vi "Close VISA Resource.vi"(8 "error in (no error)":errorcluster, 11 "Connection Info in":T1) -> (0 "error out":errorcluster)   [LabVIEW 2020, in "plugin_flodx_ph_probe.lvlib" / "plugin.lvlib" / "Instrument Manager.lvlib"]
doc: "Close the VISA resource connection. Calls mock drivers if symbol NO_DRIVER == 1."
uses:
  Instrument Manager.lvlib
  connection_info/Connection Info.ctl
  mock_driver/mock_driver.lvlib
  <instrlib>/RxnRover/FloDx Ph Probe Driver/driver_flodx_ph_probe.lvlib
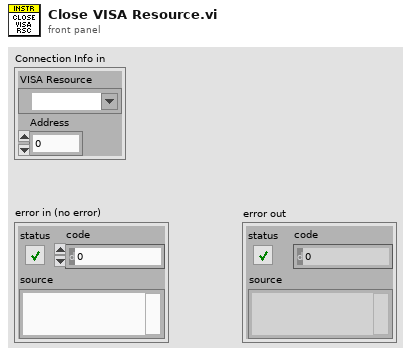
[diagram p1: front panel]
types:
  T1 = typedef "plugin_flodx_ph_probe.lvlib/plugin.lvlib/Instrument Manager.lvlib/Connection Info.ctl" = cluster{"VISA Resource":refnum<visa-resource-name>, "Address":u8}
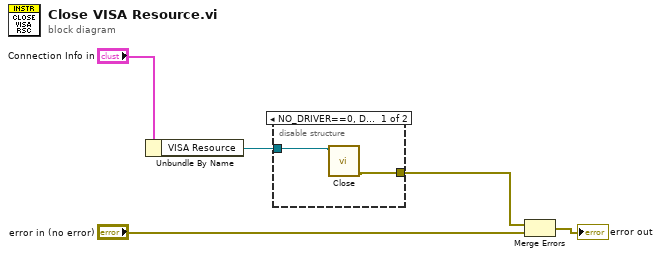
[diagram p0: block diagram]
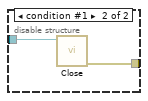
[diagram p2: hidden frame]
diagram:
  n1 = Unbundle By Name("Connection Info in") -> ("VISA Resource"=w1:refnum<visa-resource-name>)
  n2 = disable-structure shown="NO_DRIVER==0, Default" {
    disable-tunnel: [w7 w9] -> w5
    disable-tunnel: w1 -> [w6 w8]
    frame condition #0 (active) {
      n3 = call <instrlib>:"Close.vi"("VISA resource name"=w6) -> ("error out"=w7:errorcluster)  [unwired: 10 in]
    }
    frame condition #1 {
      n4 = call <instrlib>:"Close.vi"("VISA resource name"=w8) -> ("Error out"=w9:errorcluster)  [unwired: 10 in]
    }
  }
  n5 = Merge Errors(w5, "error in (no error)") -> (→"error out":errorcluster)
